vi "temp.vi"() -> ()   [LabVIEW 2024]
panel:
  in  "stop":bool
  out "green":bool
  out "yellow":bool
  out "red":bool
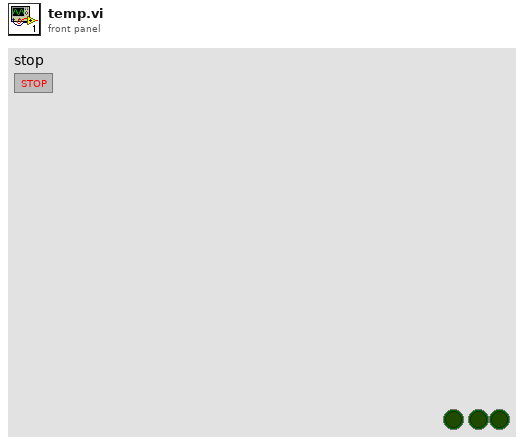
[diagram p1: front panel]
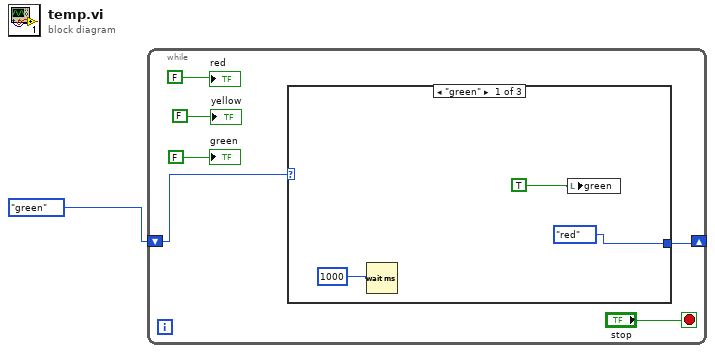
[diagram p0: block diagram]
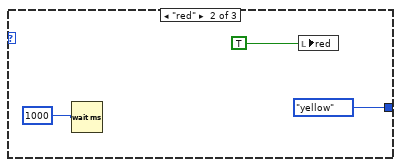
[diagram p2: hidden frame]
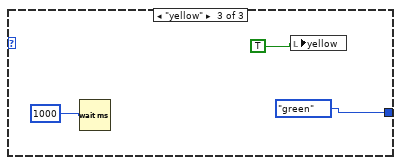
[diagram p3: hidden frame]
diagram:
  n1 = while {
    shift-right: [w4] -> _
    shift-left: enum16{"green", "yellow", "red"}."green" -> [w3]
    stop <- "stop" stop-if-true
    n2 = case shown="\"green\"" w3 {
      tunnel: [enum16{"green", "yellow", "red"}."red" enum16{"green", "yellow", "red"}."yellow" enum16{"green", "yellow", "red"}."green"] -> w4
      frame "green" {
        n3 = Wait (ms)(milliseconds to wait=u32 1000) -> ()  [unwired: 1 out]
        n4 = local write "green"(TRUE ("green")) -> ()
      }
      frame "red" {
        n5 = Wait (ms)(milliseconds to wait=u32 1000) -> ()  [unwired: 1 out]
        n6 = local write "red"(TRUE ("red")) -> ()
      }
      frame "yellow" {
        n7 = Wait (ms)(milliseconds to wait=u32 1000) -> ()  [unwired: 1 out]
        n8 = local write "yellow"(TRUE ("yellow")) -> ()
      }
    }
    "red" <- FALSE ("red")
    "yellow" <- FALSE ("yellow")
    "green" <- FALSE ("green")
  }
